vi "_Aeroflex ATT Tree.vi"   [LabVIEW 2011]
uses:
  ATT Command.ctl
panel:
  # "See Diagram"
types:
  T1 = typedef "ATT Command.ctl" = enum16{"LOAD", "INITIALIZE", "PRESET", "SET STIMULUS", "GET STIMULUS", "GET CALIBRATION", "CALIBRATE", "GET INFO", "RELEASE", "UNLOAD"}
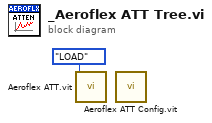
[diagram p0: block diagram]
diagram:
  n1 = call "Aeroflex ATT.vit"("ATT Command"=ATT_Command."LOAD" ("VNA Command")) -> ()  [unwired: 3 in, 8 out]
  n2 = call "Aeroflex ATT Config.vit"() -> ()  [unwired: 2 in, 10 out]
